vi "LimitMovementAmount.vi"(8 "Max rotation":dbl, 9 "Current position":dbl, 10 "Direction":bool, 11 "Move amount in":dbl) -> (1 "Movement allowed":bool, 3 "Move amount out":dbl)   [LabVIEW 2013]
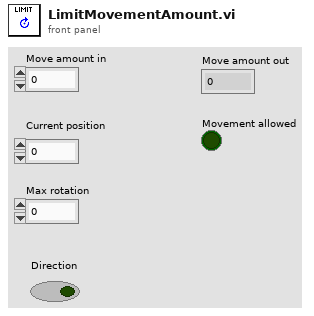
[diagram p1: front panel]
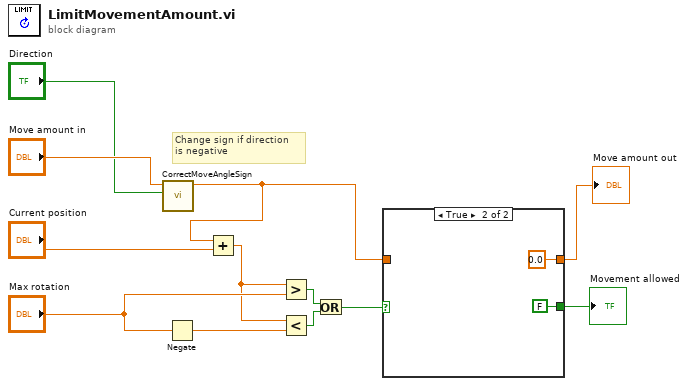
[diagram p0: block diagram]
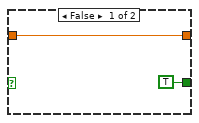
[diagram p2: hidden frame]
diagram:
  # "Change sign if direction \nis negative"
  n1 = call "CorrectMoveAngleSign.vi"("Direction"="Direction", "Step size (deg) in"="Move amount in") -> ("Step size (deg) out"=w1:dbl)  [unwired: 9 in]
  n2 = Negate(x="Max rotation") -> (-x=w9:dbl)
  n3 = Add(x=w1, y="Current position") -> (x+y=w4:dbl)
  n4 = Greater?(x=w4, y="Max rotation") -> (0:w10:bool)
  n5 = Less?(x=w4, y=w9) -> (x < y?=w11:bool)
  n6 = Or(x=w10, y=w11) -> (x .or. y?=w12:bool)
  n7 = case shown="True" w12 {
    tunnel: w1 -> [w14 _]
    tunnel: [w14 0.0 ("Wall step size (deg)")] -> w7
    tunnel: [TRUE FALSE] -> w5
    frame False {
    }
    frame True {
    }
  }
  "Move amount out" <- w7
  "Movement allowed" <- w5
